vi "Initialize MeasurementLink Session.vi"(7 "remote connection options":T2, 8 "error in":errorcluster, 9 "initialize and close session behavior":T1, 10 "session initialization parameters":T3, 11 "session factory in":refnum<class "Session Factory.lvclass">) -> (0 "error out":errorcluster, 2 "session out":variant, 3 "session factory out":refnum<class "Session Factory.lvclass">)   [LabVIEW 2021, in "NI Session Management niSE.lvlib" / "Session Factory.lvclass"]
doc: "Creates a new session using the provided <b>session initialization parameters</b>. If the session represents a remote session, <b>initialize and close session behavior</b> determines whether creating the local session creates a new session on the server or attaches to an existing session on the server."
uses:
  Session Factory.lvclass
  <vilib>/Plug-In SDKs/Sessions/Instrument/ISession Factory/Session Initialization Parameters.ctl
  <vilib>/Plug-In SDKs/Sessions/Instrument/ISession Factory/Remote Connection Options.ctl
  <vilib>/Plug-In SDKs/Sessions/Instrument/ISession Factory/Initialize and Close Session Behavior.ctl
  basic_switch_executive_driver_client/RPC Messages/nise_OpenSessionInputs.ctl
  <vilib>/Plug-In SDKs/Clients/Session Management V1/Session Reservation/Initialize and Close Session Behavior.ctl
  Session Factory.lvclass/Session Factory.ctl
  basic_switch_executive_driver_client/basic_switch_executive_driver_client.lvlib
  <vilib>/Plug-In SDKs/Clients/Session Management V1/Session Reservation/Session Reservation.lvclass
  niSE simple relay - Disconnect/SimpleSwitch/SimpleSwitchDisconnect.lvlib
  <vilib>/Plug-In SDKs/Sessions/Instrument/ISession Factory/ISession Factory.lvclass
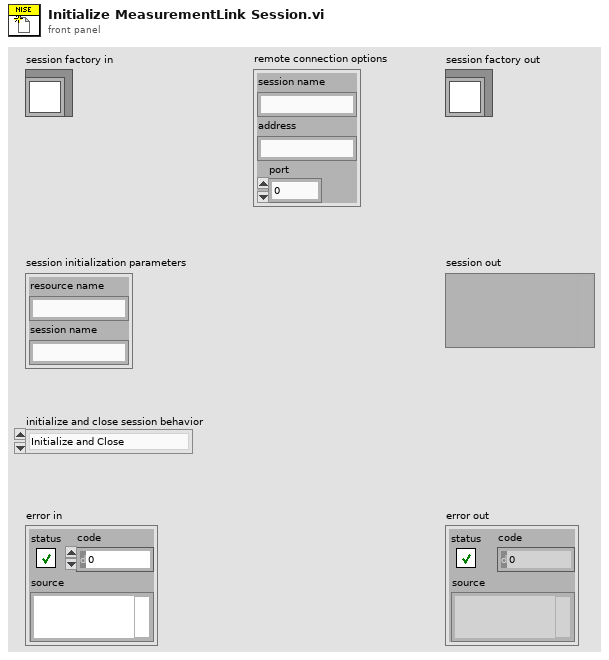
[diagram p1: front panel]
types:
  T1 = typedef "NI Session Management Instrument.lvlib/ISession Factory.lvclass/Initialize and Close Session Behavior.ctl" = enum16{"Initialize and Close", "Attach and Detach", "Initialize and Detach", "Attach and Close"}
  T2 = typedef "NI Session Management Instrument.lvlib/ISession Factory.lvclass/Remote Connection Options.ctl" = cluster{"session name":string, "address":string, "port":u32}
  T3 = typedef "NI Session Management Instrument.lvlib/ISession Factory.lvclass/Session Initialization Parameters.ctl" = cluster{"resource name":string, "session name":string}
  T4 = typedef "basic_switch_executive_driver_client.lvlib/nise_OpenSessionInputs.ctl" = cluster{"virtual_device_name":string, "optional_string":string, "initialize_and_close_session_behavior":T5}
  T5 = typedef "NI Session Management V1 Client.lvlib/Session Reservation.lvclass/Initialize and Close Session Behavior.ctl" = enum16{"Auto", "Initialize and Close", "Attach and Detach", "Initialize and Detach", "Attach and Close"}
  T6 = typedef "grpc-lvsupport-release.lvlib/grpcId.ctl" = u64
  T7 = typedef "basic_switch_executive_driver_client.lvlib/nise_SessionInformation.ctl" = cluster{"session_id":u32, "initialize_and_close_session_behavior":T5}
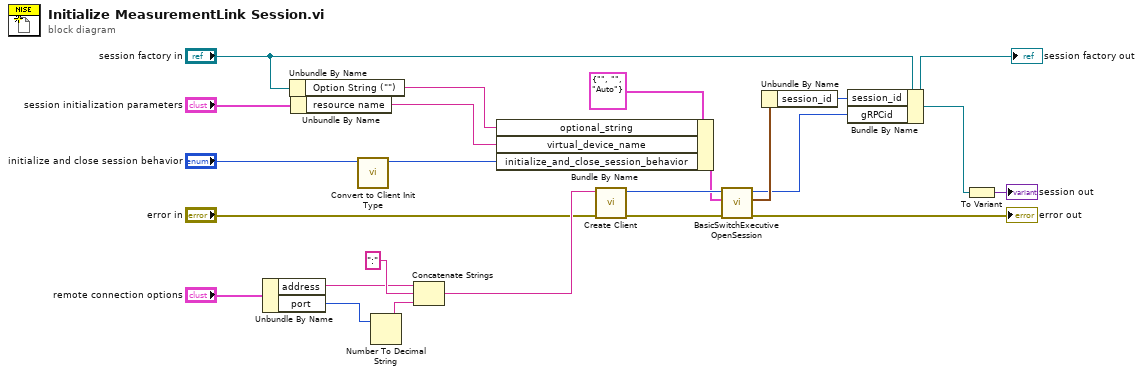
[diagram p0: block diagram]
diagram:
  n1 = Unbundle By Name("remote connection options") -> ("address"=w21:string, "port"=w20:u32)
  n2 = Unbundle By Name("session factory in") -> ("Option String (\"\")"=w7:string)
  n3 = Unbundle By Name("session initialization parameters") -> ("resource name"=w9:string)
  n4 = call "Convert to Client Init Type.vi"("initialize and close session behavior"="initialize and close session behavior") -> ("initialize_and_close_session_behavior"=w3:T5)  [unwired: 10 in]
  n5 = Number To Decimal String(number=w20) -> (decimal integer string=w19:string)  [unwired: 1 in]
  n6 = Concatenate Strings(w21, ":" ("string"), w19) -> (w18:string)
  n7 = Bundle By Name(cluster=T4 {"virtual_device_name"="", "optional_string"="", "initialize_and_close_session_behavior"=enum."Auto"} ("Request Data"), "optional_string"=w7, "virtual_device_name"=w9, "initialize_and_close_session_behavior"=w3) -> (w11:T4)
  n8 = call "Create Client.vi"("error in"="error in", "address"=w18) -> ("error out"=w16:errorcluster, "gRPC ID Out"=w17:T6)  [unwired: 8 in]
  n9 = call "BasicSwitchExecutive OpenSession.vi"("error in"=w16, "Request Data"=w11, "gRPC ID"=w17) -> ("error out"=→"error out":errorcluster, "Response Data"=w6:T7, "gRPC ID out"=w2:T6)  [unwired: 6 in]
  n10 = Unbundle By Name(w6) -> ("session_id"=w5:u32)
  n11 = Bundle By Name(cluster="session factory in", "session_id"=w5, "gRPCid"=w2) -> (w1:refnum<class "Session Factory.lvclass">)
  "session factory out" <- w1
  n12 = To Variant(anything=w1) -> (Variant=→"session out":variant)
